vi "JSON RPC Engine.vi"(8 "error in (no error)":errorcluster, 10 "methods directory":path) -> (0 "error out":errorcluster)   [LabVIEW 2020, in "JSON-RPC Lib.lvlib" / "JSONRPC Server.lvclass"]
doc: "Use this as a starting point for the RPC Server processing loop in your application"
uses:
  JSONRPC Server.lvclass
  Request/Request.lvclass/Request.ctl
  Request/request.Read method.vi
  Request/request.Read params.vi
  params/params.To JSON Tree.vi
  Add Response (Method Not Found from Request).vi
  Add Response (Result from Request).vi
  Add Response (Server Error from Request).vi
  Add Response (Internal Error from Request).vi
  Method Loader/Method Loader.lvclass
  Request/Request.lvclass
  Variant JSON API/Variant JSON API.lvlib
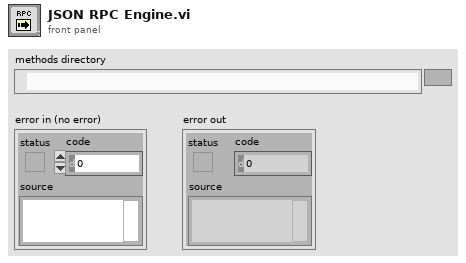
[diagram p1: front panel]
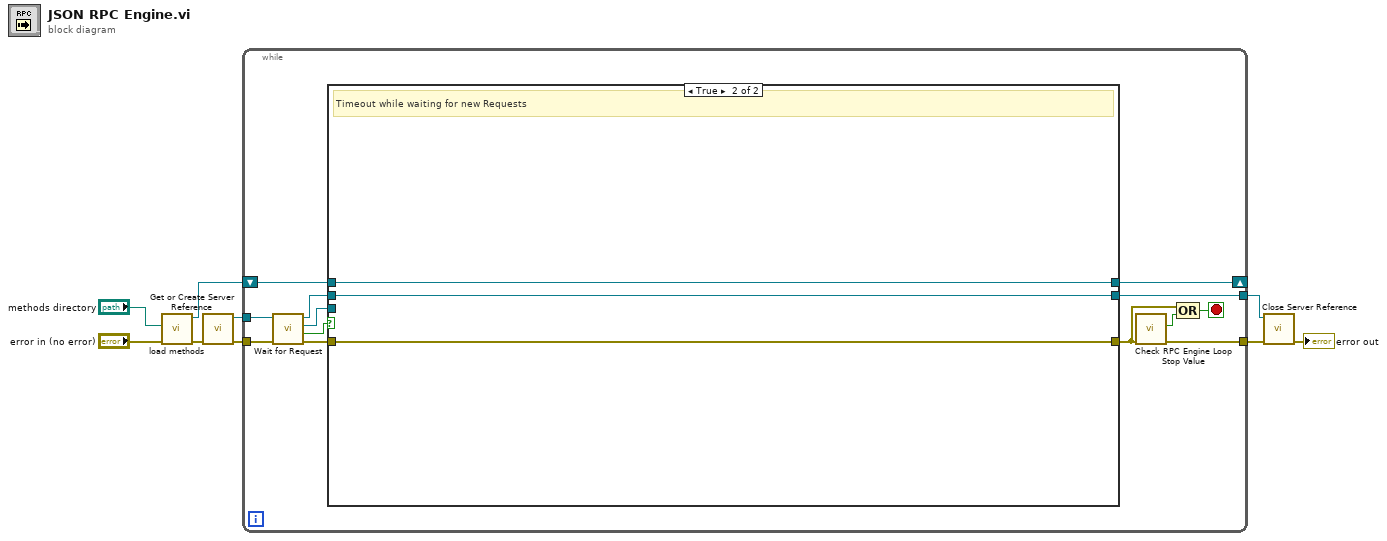
[diagram p0: block diagram]
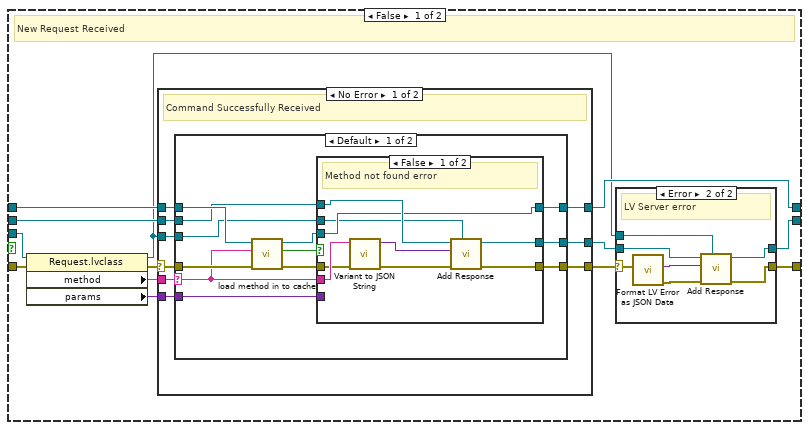
[diagram p2: hidden frame]
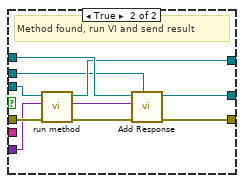
[diagram p4: hidden frame]
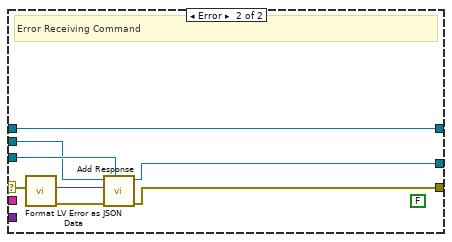
[diagram p6: hidden frame]
diagram:
  n1 = call "load methods.vi"("error in (no error)"="error in (no error)", "Folder Path"="methods directory") -> ("error out"=w5:errorcluster, "Method Manager out"=w4:refnum<class "Method Loader.lvclass">)  [unwired: 8 in]
  n2 = call "Get or Create Server Reference.vi"("error in (no error)"=w5) -> ("error out"=w8:errorcluster, "Server Out"=w9:refnum<class "JSONRPC Server.lvclass">)  [unwired: 9 in]
  n3 = while {
    tunnel: w9 -> [w22]
    tunnel: w8 -> [w18]
    tunnel: [w11] -> w6
    tunnel: [w16] -> w7
    shift-right: [w13] -> _
    shift-left: w4 -> [w14]
    stop <- w15 stop-if-true
    n4 = call "Wait for Request.vi"("error in (no error)"=w18, "Server in"=w22) -> ("error out"=w17:errorcluster, "timed out?"=w19:bool, "Request"=w20:refnum<class "Request.lvclass">, "Server out"=w21:refnum<class "JSONRPC Server.lvclass">)  [unwired: 6 in]
    n5 = case shown="True" w19 {
      tunnel: w21 -> [w30 w97]
      tunnel: w20 -> [w35 _]
      tunnel: w17 -> [w32 w98]
      tunnel: [w26 w98] -> w12
      tunnel: [w24 w97] -> w16
      tunnel: w14 -> [w29 w96]
      tunnel: [w28 w96] -> w13
      frame False {
        # "New Request Received"
        n6 = property class="Request.lvclass"(reference=w35, error in=w32) -> (reference out=w23:refnum<class "Request.lvclass">, error out=w31:errorcluster, "method"=w34:string, "params"=w33:variant)
        n7 = case shown="No Error" w31 {
          selector: w31 -> [w51 w90]
          tunnel: w34 -> [w53 _]
          tunnel: w33 -> [w45 _]
          tunnel: [w48 w92] -> w27
          tunnel: w30 -> [w50 w94]
          tunnel: [w47 w93] -> w25
          tunnel: w23 -> [w46 w95]
          tunnel: w29 -> [w52 w88]
          tunnel: [w49 w88] -> w28
          frame No Error {
            # "Command Successfully Received"
            n8 = case shown="Default" w53 {
              selector: w53 -> [w55 _]
              tunnel: w52 -> [w65 w87]
              tunnel: w51 -> [w61 w86]
              tunnel: w50 -> [w60 w85]
              tunnel: [w59 w87] -> w49
              tunnel: [w57 w86] -> w48
              tunnel: [w58 w85] -> w47
              tunnel: w46 -> [w56 _]
              tunnel: w45 -> [w54 _]
              frame Default {
                n9 = call "load method in to cache.vi"("error in (no error)"=w61, "method name"=w55, "Method Manager in"=w65) -> ("error out"=w62:errorcluster, "found?"=w64:bool, "Method Manager out"=w63:refnum<class "Method Loader.lvclass">)  [unwired: 6 in]
                n10 = case shown="False" w64 {
                  tunnel: w63 -> [w67 w84]
                  tunnel: w62 -> [w73 w83]
                  tunnel: w60 -> [w71 w82]
                  tunnel: [w67 w79] -> w59
                  tunnel: [w70 w77] -> w58
                  tunnel: [w68 w78] -> w57
                  tunnel: w56 -> [w66 w76]
                  tunnel: w55 -> [w74 _]
                  tunnel: w54 -> [_ w75]
                  frame False {
                    # "Method not found error"
                    n11 = call "Variant to JSON String.vi"("error in (no error)"=w73, "Variant in"=w74) -> ("error out"=w69:errorcluster, "Variant out"=w72:variant)  [unwired: 7 in, 1 out]
                    n12 = call-poly "Add Response.vi"("Request"=w66, "error in (no error)"=w69, "data"=w72, "Server in"=w71) -> ("error out"=w68:errorcluster, "Server out"=w70:refnum<class "JSONRPC Server.lvclass">)  [unwired: 5 in, 1 out]
                  }
                  frame True {
                    # "Method found, run VI and send result"
                    n13 = call "run method.vi"("error in (no error)"=w83, "JSON Value in"=w75, "Method Manager in"=w84) -> ("error out"=w81:errorcluster, "JSON Value out"=w80:variant, "Method Manager out"=w79:refnum<class "Method Loader.lvclass">)  [unwired: 6 in]
                    n14 = call-poly "Add Response.vi"("Request"=w76, "error in (no error)"=w81, "JSON Value in"=w80, "Server in"=w82) -> ("error out"=w78:errorcluster, "Server out"=w77:refnum<class "JSONRPC Server.lvclass">)  [unwired: 5 in, 1 out]
                  }
                }
              }
              frame "shutdown_rpc_server" {
              }
            }
          }
          frame Error {
            (unwired) FALSE
            # "Error Receiving Command"
            n15 = call "Format LV Error as JSON Data.vi"("error in"=w90) -> ("error out"=w91:errorcluster, "Error Value out"=w89:variant)  [unwired: 9 in]
            n16 = call-poly "Add Response.vi"("Request"=w95, "error in (no error)"=w91, "data"=w89, "Server in"=w94) -> ("error out"=w92:errorcluster, "Server out"=w93:refnum<class "JSONRPC Server.lvclass">)  [unwired: 5 in, 1 out]
          }
        }
        n17 = case shown="Error" w27 {
          selector: w27 -> [w37 w40]
          tunnel: [w37 w39] -> w26
          tunnel: w25 -> [w36 w43]
          tunnel: [w36 w42] -> w24
          tunnel: w23 -> [_ w38]
          frame No Error {
          }
          frame Error {
            # "LV Server error"
            n18 = call "Format LV Error as JSON Data.vi"("error in"=w40) -> ("error out"=w41:errorcluster, "Error Value out"=w44:variant)  [unwired: 9 in]
            n19 = call-poly "Add Response.vi"("Request"=w38, "error in (no error)"=w41, "data"=w44, "Server in"=w43) -> ("error out"=w39:errorcluster, "Server out"=w42:refnum<class "JSONRPC Server.lvclass">)  [unwired: 5 in, 1 out]
          }
        }
      }
      frame True {
        # "Timeout while waiting for new Requests"
      }
    }
    n20 = call "Check RPC Engine Loop Stop Value.vi"("error in (no error)"=w12) -> ("error out"=w11:errorcluster, "stopped?"=w10:bool)  [unwired: 9 in]
    n21 = Compound Arithmetic op=OR(w12, w10) -> (w15:bool)
  }
  n22 = call "Close Server Reference.vi"("error in (no error)"=w6, "Server in"=w7) -> ("error out"=→"error out":errorcluster)  [unwired: 9 in]
